vi "algo2.vi"() -> ()   [LabVIEW 2015]
uses:
  <vilib>/vision/NI_Vision_Development_Module.lvlib
panel:
  in  "Color Mode":u16(ring) items=["RGB", "HSL", "HSV", "HSI"]
  out "error out 2":errorcluster
  out "Red or Hue Plane out":T1(plugin-control)
  in  "stop":bool
  out "Image Out":T1(plugin-control)
  out "error out":errorcluster
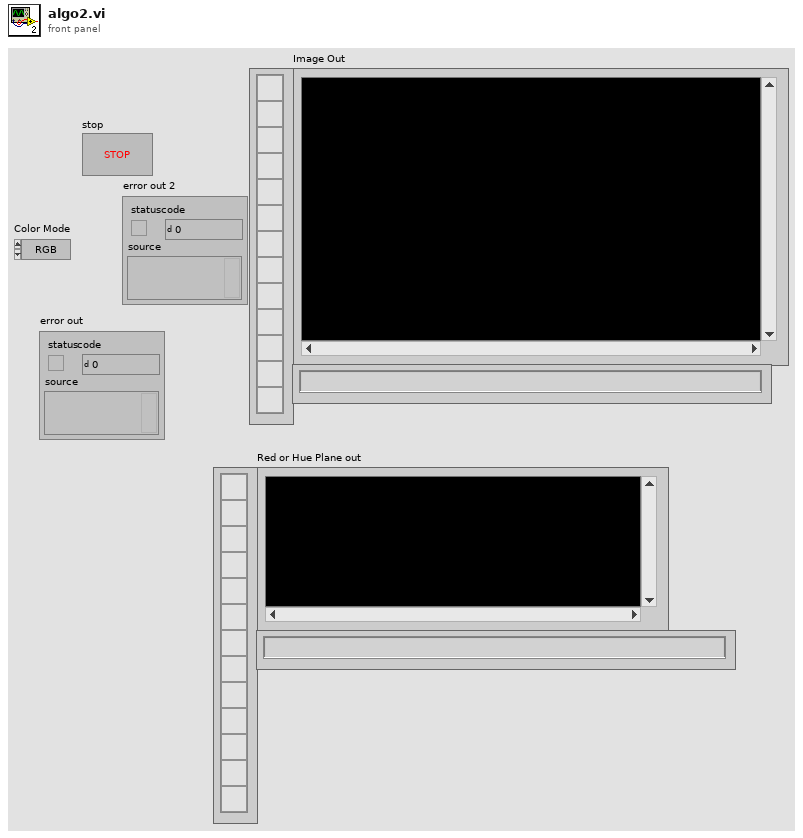
[diagram p1: front panel]
types:
  T1 = typedef "IMAQ Image.ctl" = refnum<image>
  T2 = typedef "Image Type" = u32
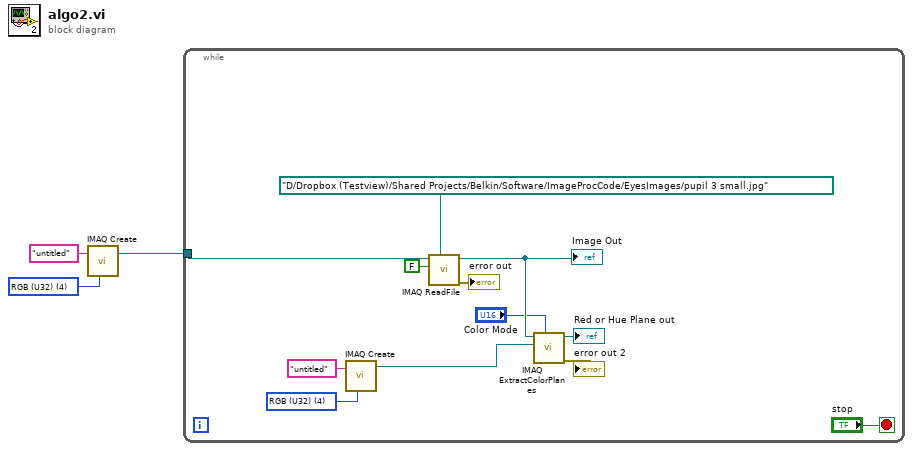
[diagram p0: block diagram]
diagram:
  w3 = T2 4 items=["Grayscale (U8)", "Grayscale (I16)", "Grayscale (SGL)", "Complex (CSG)", "RGB (U32)", "HSL (U32)", "RGB (U64)", "Grayscale (U16)"] ("Image Type")
  n1 = call "IMAQ Create"("Image Name"="untitled", "Image Type"=w3) -> ("New Image"=w1:T1)  [unwired: 2 in, 2 out]
  n2 = while {
    tunnel: w1 -> [w13]
    stop <- "stop" stop-if-true
    w7 = T2 4 items=["Grayscale (U8)", "Grayscale (I16)", "Grayscale (SGL)", "Complex (CSG)", "RGB (U32)", "HSL (U32)", "RGB (U64)", "Grayscale (U16)"] ("Image Type")
    n3 = call "IMAQ Create"("Image Name"="untitled", "Image Type"=w7) -> ("New Image"=w5:T1)  [unwired: 2 in, 2 out]
    n4 = call "IMAQ ReadFile"("File Path"=path "D:/Dropbox (Testview)/Shared Projects/Belkin/Software/ImageProcCode/EyesImages/pupil 3 small.jpg", "Load Color Palette? (No)"=FALSE, "Image"=w13) -> ("error out"=→"error out":errorcluster, "Image Out"=w10:T1)  [unwired: 4 in, 3 out]
    "Image Out" <- w10
    n5 = call "IMAQ ExtractColorPlanes"("Color Mode"="Color Mode", "Red or Hue Plane"=w5, "Image Src"=w10) -> ("error out"=→"error out 2":errorcluster, "Red or Hue Plane out"=→"Red or Hue Plane out":T1)  [unwired: 5 in, 2 out]
  }
